vi "82CallSystemForms.vi"(2 "error in (no error)":errorcluster, 3 "OK Button":bool) -> (0 "error out":errorcluster, 1 "ButtonPressed":i32(ring) items=["None", "OK", "Cancel", "Abort", "Retry", "Ignore", "Yes", "No"], 4 "Path":path)   [LabVIEW 2014]
uses:
  System.Windows.Forms
panel:
  # "NOTE:"
  # "File » VI Properties,,, » Execution » Preferred Execution System: user interface"
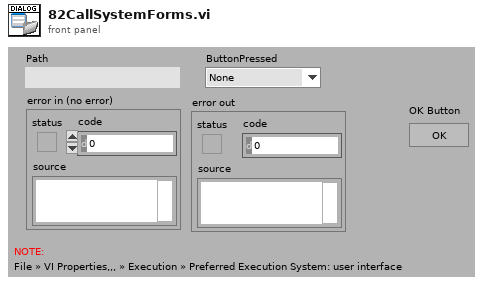
[diagram p1: front panel]
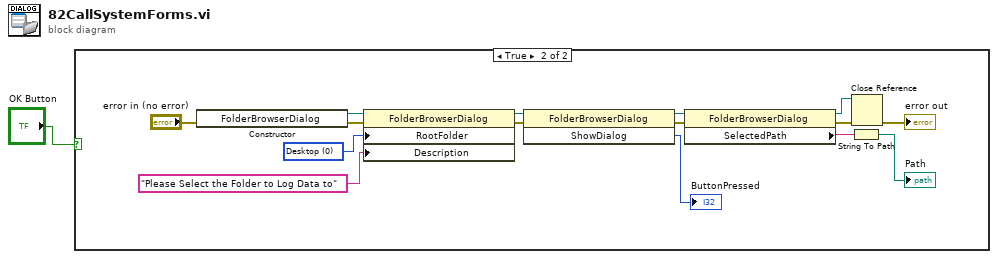
[diagram p0: block diagram]
diagram:
  n1 = case shown="True" "OK Button" {
    frame False {
    }
    frame True {
      w14 = 0 items=["Desktop"=0, "Programs"=2, "Personal, MyDocuments"=5, "Favorites"=6, "Startup"=7, "Recent"=8, "SendTo"=9, "StartMenu"=11, "MyMusic"=13, "DesktopDirectory"=16, "MyComputer"=17, "Templates"=21, "ApplicationData"=26, "LocalApplicationData"=28, "InternetCache"=32, "Cookies"=33, "History"=34, "CommonApplicationData"=35, "System"=37, "ProgramFiles"=38, "MyPictures"=39, "CommonProgramFiles"=43] ("RootFolder")
      n2 = constructor class="FolderBrowserDialog"(error in="error in (no error)") -> (reference out=w16:refnum<k24>, error out=w15:errorcluster)  [unwired: 2 in, 1 out]
      n3 = property class="FolderBrowserDialog"(reference=w16, error in=w15, "RootFolder"=w14, "Description"="Please Select the Folder to Log Data to") -> (reference out=w12:refnum<k24>, error out=w11:errorcluster)
      n4 = invoke class="FolderBrowserDialog" method="ShowDialog"(reference=w12, error in=w11) -> (reference out=w10:refnum<k24>, error out=w9:errorcluster, "ShowDialog"=→"ButtonPressed":i32)  [unwired: 1 in]
      n5 = property class="FolderBrowserDialog"(reference=w10, error in=w9) -> (reference out=w6:refnum<k24>, error out=w7:errorcluster, "SelectedPath"=w8:string)
      n6 = String To Path(string=w8) -> (path=→"Path":path)
      n7 = Close Reference(reference=w6, error in (no error)=w7) -> (error out=→"error out":errorcluster)
    }
  }
